vi "compress.vi"(7 "compressionLevel":i32, 8 "错误输入（无错误）":errorcluster, 11 "src":string) -> (0 "错误输出":errorcluster, 3 "dst":string)   [LabVIEW 2020, in "zstd.lvlib"]
uses:
  zstd.lvlib
  libzstd.dll
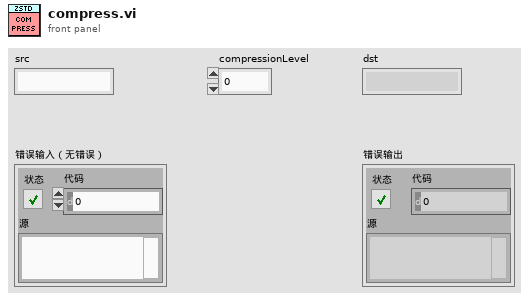
[diagram p1: front panel]
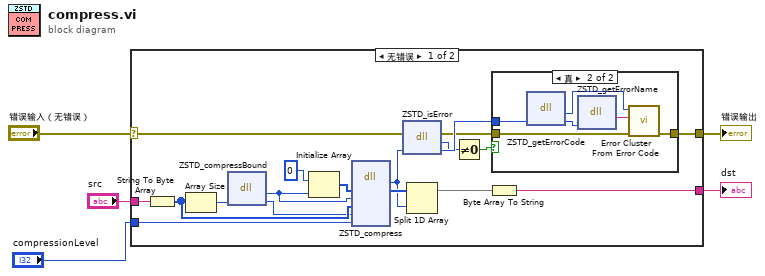
[diagram p0: block diagram]
diagram:
  n1 = case shown="无错误" "错误输入（无错误）" {
    selector: "错误输入（无错误）" -> [w7 w31]
    tunnel: "src" -> [w19 _]
    tunnel: [w16 _] -> w3
    tunnel: [w13 w31] -> w5
    tunnel: "compressionLevel" -> [w8 _]
    frame No Error {
      n2 = String To Byte Array(string=w19) -> (unsigned byte array=w18:u8[])
      n3 = Array Size(array=w18) -> (size(s)=w21:i32)
      n4 = dll-call lib="D:/Workspace/LabVIEW/LVToolset/vi.lib/zstd/libzstd.dll" fn="ZSTD_compressBound"("srcSize"=w21) -> ("return"=w10:u32, "srcSize"=w9:u32)  [unwired: 3 in, 2 out]
      n5 = Initialize Array(u8 0 ("无符号8位整型"), w10) -> (w22:u8[])
      n6 = dll-call lib="D:/Workspace/LabVIEW/LVToolset/vi.lib/zstd/libzstd.dll" fn="ZSTD_compress"("dst"=w22, "dstCapacity"=w10, "src"=w18, "srcSize"=w9, "compressionLevel"=w8) -> ("return"=w15:u32, "dst"=w20:u8[])  [unwired: 7 in, 2 out]
      n7 = dll-call lib="D:/Workspace/LabVIEW/LVToolset/vi.lib/zstd/libzstd.dll" fn="ZSTD_isError"(error in=w7, "result"=w15) -> (error out=w6:errorcluster, "return"=w12:u8, "result"=w14:u32)  [unwired: 2 in, 1 out]
      n8 = Split 1D Array(array=w20, index=w15) -> (first subarray=w17:u8[])  [unwired: 1 out]
      n9 = Not Equal To 0?(x=w12) -> (x != 0?=w11:bool)
      n10 = Byte Array To String(unsigned byte array=w17) -> (string=w16:string)
      n11 = case shown="真" w11 {
        tunnel: w14 -> [_ w30]
        tunnel: [w24 w26] -> w13
        tunnel: w6 -> [w24 w25]
        frame False {
        }
        frame True {
          n12 = dll-call lib="D:/Workspace/LabVIEW/LVToolset/vi.lib/zstd/libzstd.dll" fn="ZSTD_getErrorCode"("functionResult"=w30) -> ("return"=w27:i32, "functionResult"=w29:u32)  [unwired: 3 in, 2 out]
          n13 = dll-call lib="D:/Workspace/LabVIEW/LVToolset/vi.lib/zstd/libzstd.dll" fn="ZSTD_getErrorName"("code"=w29) -> ("return"=w28:string)  [unwired: 4 in, 2 out]
          n14 = call <vilib>:"Error Cluster From Error Code.vi"("error in (no error)"=w25, "error message (\"\")"=w28, "error code (0)"=w27) -> ("error out"=w26:errorcluster)  [unwired: 6 in]
        }
      }
    }
    frame Error {
    }
  }
  "错误输出" <- w5
  "dst" <- w3
